vi "ELVIS III v1.0 Unreserve Encoder.vi"(7 "Allow multiple opens?":bool, 8 "error in (no error)":errorcluster, 10 "Encoder Channel":T2, 11 "myRIO FPGA Ref Out":T1) -> (0 "error out":errorcluster)   [LabVIEW 2021]
uses:
  <vilib>/myRIO/Common/Instrument Driver Framework/myRIO v1.0/Encoder/typedefs/Encoder Channels Enum.ctl
  <vilib>/myRIO/Common/Instrument Driver Framework/Utilities/typedefs/Generic FPGA Reference.ctl
  <vilib>/myRIO/Common/Instrument Driver Framework/ELVIS III v1.0/Resource Manager/vis/ELVIS III v1.0 Create Configuration List.vi
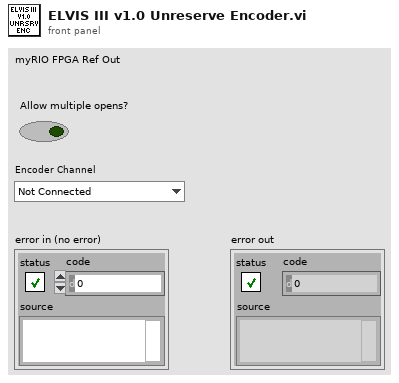
[diagram p1: front panel]
types:
  T1 = typedef "Generic FPGA Reference.ctl" = refnum<k20>
  T2 = typedef "Encoder Channels Enum.ctl" = enum16{"Not Connected", "C/ENC0", "C/ENC1", "A/ENC", "A/ENC0", "A/ENC1", "A/ENC2", "A/ENC3", "A/ENC4", "A/ENC5", "A/ENC6", "A/ENC7", "A/ENC8", "A/ENC9", "B/ENC", "B/ENC0", "B/ENC1", "B/ENC2", "B/ENC3", "B/ENC4", "B/ENC5", "B/ENC6", "B/ENC7", "B/ENC8", "B/ENC9", "DIO/ENC0", "DIO/ENC1", "DIO/ENC2", "DIO/ENC3", "DIO/ENC4"}
  T3 = typedef "ELVIS III v1.0 Channel Reservation List.ctl" = T4[]
  T4 = typedef "ELVIS III v1.0 Channel Reservation Info.ctl" = cluster{"Channel Name":string, "Connector":T5, "MutexIDs":u32[]}
  T5 = typedef "ELVIS III v1.0 Connector List.ctl" = enum32{"None", "ConnectorA", "ConnectorB"}
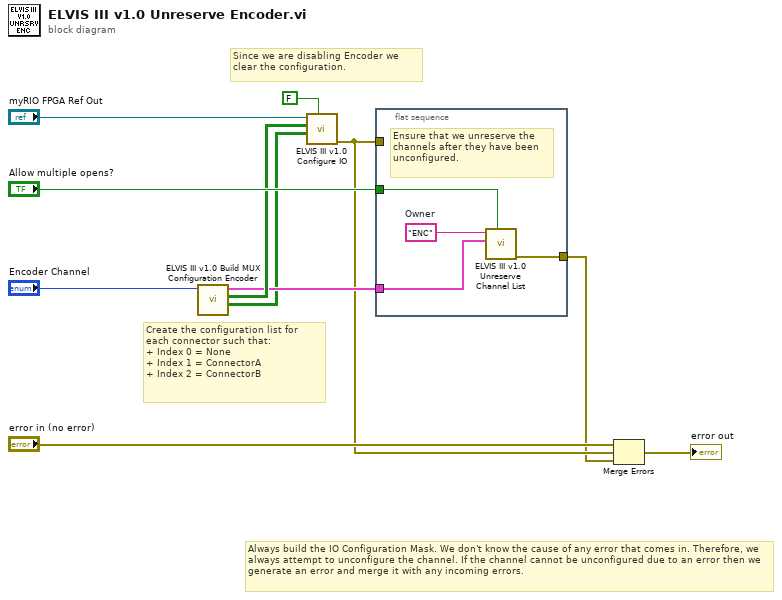
[diagram p0: block diagram]
diagram:
  # "Since we are disabling Encoder we clear the configuration."
  # "Always build the IO Configuration Mask. We don't know the cause of any error that comes in. Therefore, we always attempt to unconfigure the channel. If the channel cannot be unconfigured due to an error then we generate an error and merge it with any incoming errors."
  # "Create the configuration list for each connector such that:\n+ Index 0 = None\n+ Index 1 = ConnectorA\n+ Index 2 = ConnectorB"
  n1 = call <vilib>:"ELVIS III v1.0 Build MUX Configuration Encoder.vi"("Channel"="Encoder Channel") -> ("Configuration Bitmask Array"=w1:bool[][], "Configuration BitCode Array"=w5:bool[][], "Channel Reservation List"=w4:T3)  [unwired: 8 in]
  n2 = call <vilib>:"ELVIS III v1.0 Configure IO.vi"("Value"=FALSE ("Clear?"), "Bitmask Array"=w1, "Bitcode Array"=w5, "myRIO FPGA Ref In"="myRIO FPGA Ref Out") -> ("error out"=w3:errorcluster)  [unwired: 7 in]
  n3 = flat-sequence {
    tunnel: "Allow multiple opens?" -> [w15]
    tunnel: w4 -> [w13]
    tunnel: w3 -> [_]
    tunnel: [w12] -> w2
    frame #0 {
      w14 = "ENC"  # Owner
      # "Ensure that we unreserve the channels after they have been unconfigured."
      n4 = call <vilib>:"ELVIS III v1.0 Unreserve Channel List.vi"("Allow multiple opens?"=w15, "Channel Reservation List"=w13, "Owner"=w14) -> ("error out"=w12:errorcluster)  [unwired: 8 in]
    }
  }
  n5 = Merge Errors("error in (no error)", w3, w2) -> (→"error out":errorcluster)
